vi "Get SMO Port.vi"(8 "error in (no error)":errorcluster, 11 "Inst.MOTORInstrument in":refnum<class "Inst.MOTOR.lvclass">) -> (0 "error out":errorcluster, 2 "Port":u16, 3 "Inst.MOTORInstrument out":refnum<class "Inst.MOTOR.lvclass">)   [LabVIEW 2019, in "Inst.MOTOR.lvclass"]
uses:
  Inst.MOTOR.lvclass
  <userlib>/Levylab/Instrument Framework/Instrument Types/VSource/Instrument.VSource.lvclass
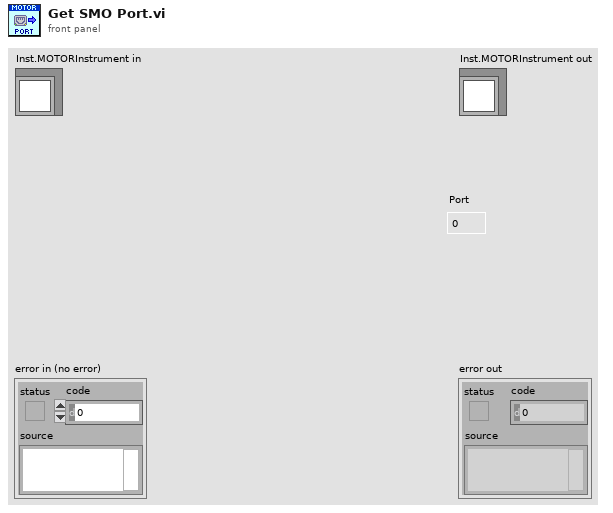
[diagram p1: front panel]
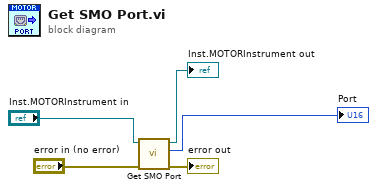
[diagram p0: block diagram]
diagram:
  n1 = call-parent "Get SMO Port.vi"("error in (no error)"="error in (no error)", "Instrument in"="Inst.MOTORInstrument in") -> ("error out"=→"error out":errorcluster, "Port"=→"Port":u16, "Instrument out"=→"Inst.MOTORInstrument out":refnum<class "Inst.MOTOR.lvclass">)  [unwired: 7 in]
